vi "ex_Wire Controls to ConPane.vi"(8 "error in (no error)":errorcluster, 9 "All Controls":string[](array[string]), 10 "Controls to Wire":string[](array[string]), 11 "VI refnum in":refnum<vi>) -> (0 "Error Out":errorcluster, 2 "Controls[]":refnum<vi>[](array[refnum]), 3 "VI refnum out":refnum<vi>)   [LabVIEW 2020]
doc: "Wires controls of front panel specified by the VI refnum in to its connector pane. You wire in a list of names of all the available controls and a list of names of the controls you want wired to the connector pane. The VI refnum is returned as well as the control refnums for all the controls on the VI's front panel."
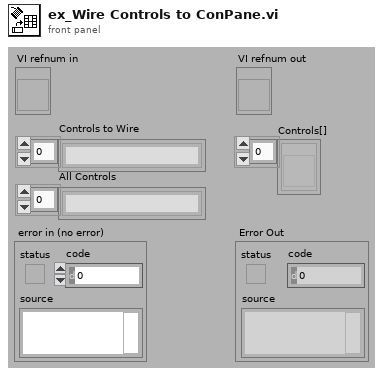
[diagram p1: front panel]
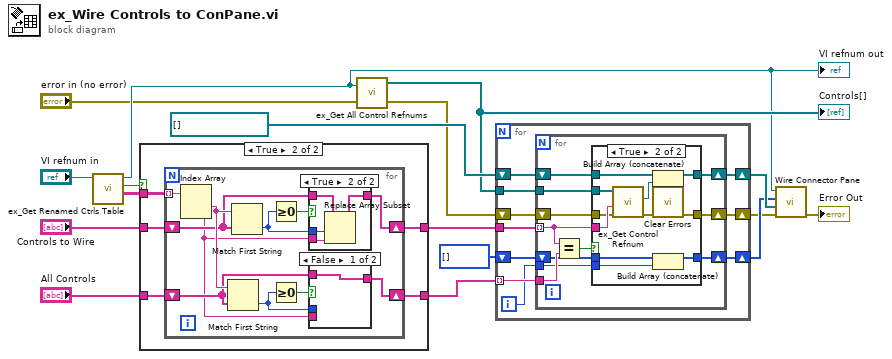
[diagram p0: block diagram]
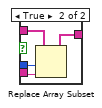
[diagram p4: hidden frame]
diagram:
  n1 = call <vilib>:"ex_Get Renamed Ctrls Table.vi"("VI refnum"="VI refnum in") -> ("Renamed Controls"=w9:string[][], "Tag available?"=w10:bool, "VI refnum out"=w2:refnum<vi>)  [unwired: 7 in, 1 out]
  "VI refnum out" <- w2
  n2 = case shown="True" w10 {
    tunnel: w9 -> [_ w22]
    tunnel: [w18 w23] -> w8
    tunnel: "Controls to Wire" -> [w18 w21]
    tunnel: [w17 w20] -> w5
    tunnel: "All Controls" -> [w17 w19]
    frame False {
    }
    frame True {
      n3 = for {
        tunnel: w22 -> [w34] mode=indexing
        shift-right: [w32] -> w23
        shift-left: w21 -> [w31]
        shift-right: [w26] -> w20
        shift-left: w19 -> [w25]
        n4 = Index Array(array=w34) -> (element #1=w33:string, element #2=w24:string)  [unwired: 2 in]
        n5 = Match First String(2:w25, 3:w33) -> (0:w27:i32)  [unwired: 1 out]
        n6 = Match First String(2:w31, 3:w33) -> (0:w30:i32)  [unwired: 1 out]
        n7 = Greater Or Equal To 0?(x=w30) -> (x >= 0?=w28:bool)
        n8 = Greater Or Equal To 0?(x=w27) -> (x >= 0?=w29:bool)
        n9 = case shown="True" w28 {
          tunnel: w31 -> [w35 w39]
          tunnel: w30 -> [_ w38]
          tunnel: [w35 w37] -> w32
          tunnel: w24 -> [_ w36]
          frame False {
          }
          frame True {
            n10 = Replace Array Subset(array=w39, new element=w36, index=w38) -> (w37:string[])
          }
        }
        n11 = case shown="False" w29 {
          tunnel: w25 -> [w40 w44]
          tunnel: w27 -> [_ w43]
          tunnel: [w40 w42] -> w26
          tunnel: w24 -> [_ w41]
          frame False {
          }
          frame True {
            n12 = Replace Array Subset(array=w44, new element=w41, index=w43) -> (w42:string[])
          }
        }
      }
    }
  }
  n13 = call <vilib>:"ex_Get All Control Refnums.vi"("viref Express VI"=w2) -> ("All Controls[]"=w3:refnum<vi>[])  [unwired: 2 in, 1 out]
  "Controls[]" <- w3
  n14 = for {
    tunnel: w3 -> [w52]
    tunnel: w8 -> [w53]
    tunnel: w5 -> [w54] mode=indexing
    shift-right: [w45] -> w16
    shift-left: refnum<vi>[] [] ("Array of refnums in") -> [w46]
    shift-right: [w47] -> w15
    shift-left: i32[] [] -> [w48]
    shift-right: [w49] -> w14
    shift-left: "error in (no error)" -> [w50]
    i -> [w51]
    n15 = for {
      tunnel: w54 -> [w65]
      tunnel: w53 -> [w62] mode=indexing
      tunnel: w52 -> [w63]
      tunnel: w51 -> [w61]
      shift-right: [w60] -> w49
      shift-left: w50 -> [w59]
      shift-right: [w58] -> w47
      shift-left: w48 -> [w57]
      shift-right: [w56] -> w45
      shift-left: w46 -> [w55]
      n16 = Equal?(x=w62, y=w65) -> (x = y?=w64:bool)
      n17 = case shown="True" w64 {
        tunnel: w63 -> [_ w79]
        tunnel: w62 -> [_ w78]
        tunnel: [w68 w76] -> w56
        tunnel: w55 -> [w68 w75]
        tunnel: w57 -> [w67 w74]
        tunnel: [w67 w73] -> w58
        tunnel: w61 -> [_ w72]
        tunnel: [w66 w69] -> w60
        tunnel: w59 -> [w66 w71]
        frame False {
        }
        frame True {
          n18 = call <vilib>:"ex_Get Control Refnum.vi"("error in (no error)"=w71, "Name"=w78, "Controls[]"=w79) -> ("error out"=w70:errorcluster, "Ctl Refnum"=w77:refnum<vi>)  [unwired: 7 in]
          n19 = Build Array (concatenate)(w75, w77) -> (w76:refnum<vi>[])
          n20 = call <vilib>:"Clear Errors.vi"("error in (no error)"=w70) -> ("error out"=w69:errorcluster)  [unwired: 5 in, 1 out]
          n21 = Build Array (concatenate)(w74, w72) -> (w73:i32[])
        }
      }
    }
  }
  n22 = call <vilib>:"Wire Connector Pane.vi"("Error In"=w14, "Controls"=w16, "Control Indices"=w15, "VI refnum"=w2) -> ("Error Out"=→"Error Out":errorcluster)  [unwired: 7 in]
